vi "File is Open.vi"(8 "error in (no error)":errorcluster, 11 "Mock Configurable Base in":refnum<class "Mock Configurable Base.lvclass">) -> (0 "error out":errorcluster, 2 "Is open?":bool, 3 "Mock Configurable Base out":refnum<class "Mock Configurable Base.lvclass">)   [LabVIEW 2020, in "Mock Configurable Base.lvclass"]
uses:
  Mock Configurable Base.lvclass
  Mock Configurable Base.lvclass/Mock Configurable Base.ctl
  <vilib>/Utility/config.llb/Config Data RefNum.ctl
  <vilib>/Utility/config.llb/NI_LVConfig.lvlib
  source/Framework/Configuration/Configuration.lvclass
  C:/Git/astemes-triarc-framework/source/Framework/Base/Base.lvclass
  C:/Git/astemes-triarc-framework/source/Framework/Configuration File/Configuration File.lvclass
  C:/Git/astemes-triarc-framework/source/Framework/Configuration/Configuration.lvclass
  C:/Git/astemes-triarc-framework/tests/Mock Configurable Base/Mock Configurable Base.lvclass
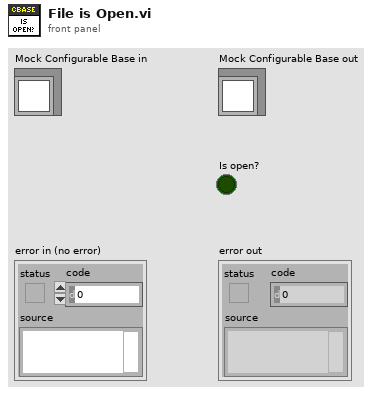
[diagram p1: front panel]
types:
  T1 = typedef "NI_LVConfig.lvlib/Config Data RefNum.ctl" = refnum<k1>
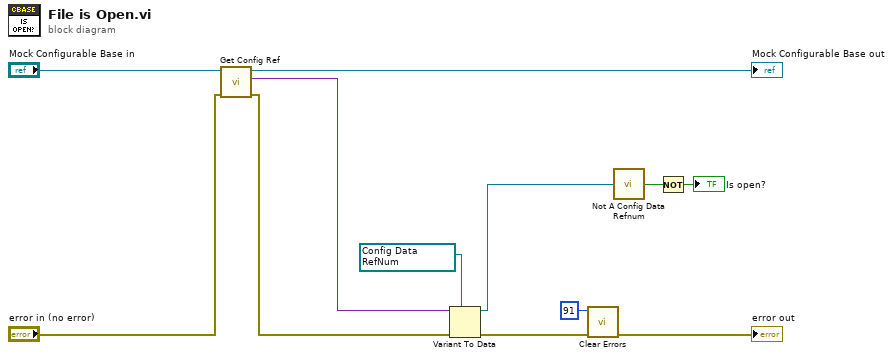
[diagram p0: block diagram]
diagram:
  w10 = T1 refnum items=["config data"] ("refnum out")
  n1 = call "Get Config Ref.vi"("error in (no error)"="error in (no error)", "Configuration In"="Mock Configurable Base in") -> ("error out"=w11:errorcluster, "Reference"=w12:variant, "Configuration Out"=→"Mock Configurable Base out":refnum<class "Mock Configurable Base.lvclass">)  [unwired: 7 in]
  n2 = Variant To Data(error in=w11, type=w10, Variant=w12) -> (data=w3:T1, error out=w9:errorcluster)
  n3 = call <vilib>:"Clear Errors.vi"("error in (no error)"=w9, "specific error code to clear (0: all)"=91) -> ("error out"=→"error out":errorcluster)  [unwired: 4 in, 1 out]
  n4 = call <vilib>:"Not A Config Data Refnum.vi"("refnum"=w3) -> ("not a config data refnum"=w2:bool)
  n5 = Not(x=w2) -> (.not. x?=→"Is open?":bool)
